vi "Main.vi"() -> ()   [LabVIEW 2018]
panel:
  out "Waveform Graph":dbl[](graph)
  out "error out":errorcluster {"code" format="%.0x"}
  in  "Channel Name (\"CH1\")":string="ch1"
  in  "resource name":refnum<k15>
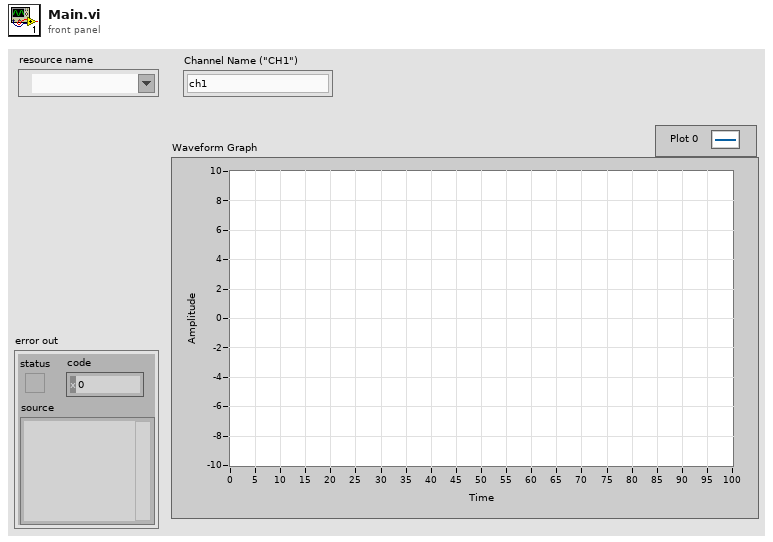
[diagram p1: front panel]
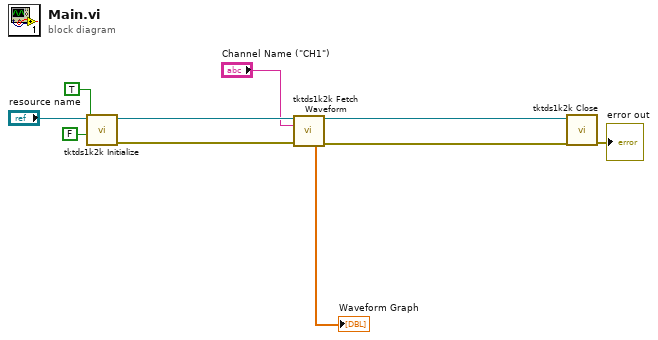
[diagram p0: block diagram]
diagram:
  n1 = call <instrlib>:"tktds1k2k Initialize.vi"("Reset Device (Yes)"=FALSE, "ID Query (Yes)"=TRUE, "resource name"="resource name") -> ("error out"=w8:errorcluster, "instrument handle out"=w9:refnum<k15>)  [unwired: 7 in]
  n2 = call <instrlib>:"tktds1k2k Fetch Waveform.vi"("instrument handle"=w9, "Channel Name (\"CH1\")"="Channel Name (\"CH1\")", "error in (no error)"=w8) -> ("instrument handle out"=w4:refnum<k15>, "Waveform Array"=→"Waveform Graph":dbl[], "error out"=w3:errorcluster)  [unwired: 7 in, 3 out]
  n3 = call <instrlib>:"tktds1k2k Close.vi"("error in (no error)"=w3, "instrument handle"=w4) -> ("error out"=→"error out":errorcluster)  [unwired: 9 in]
